vi "CAN Communication.vi"(8 "error in":errorcluster) -> (0 "error out":errorcluster)   [LabVIEW 2016]
uses:
  Typedefs/CAN Refnum.ctl
  Typedefs/CAN Session Pointer.ctl
  Typedefs/CAN Communication References.ctl
  Typedefs/kill process notifier array.ctl
  Typedefs/Write Queue.ctl
  Typedefs/FPGA CAN Frame Cluster.ctl
  <vilib>/userdefined/High Color/nirio_resource_hc.ctl
  <vilib>/FPGAPlugInAG/cRIO-9033/niLvFpga_Open_cRIO-9033.vi
  <vilib>/Utility/error.llb/Error Cluster From Error Code.vi
  <vilib>/RVI Host/nirviSupport.llb/nirviErrorClusterFromErrorCode.vi
  <vilib>/rvi/errors/niLvFpgaAdjustHostInterfaceError.vi
  <vilib>/FPGAPlugInAG/cRIO-9033/niLvFpga_Close_cRIO-9033.vi
  <vilib>/rvi/interface/nirviOpenFPGA/nirviOpenFPGA.xnode
  Users/s163601/Desktop/05-28/FPGA Bitfiles/project_FPGATarget_FPGAMain_boaNRF5GBP4.lvbitx
  Users/s163601/Desktop/05-28/FPGA Main.vi
  <vilib>/rvi/interface/nirviMethod/nirviMethod.xnode
  <vilib>/rvi/interface/nirviReadWriteControl/nirviReadWriteControl.xnode
  <vilib>/rvi/interface/nirviCloseFPGA/nirviCloseFPGA.xnode
  NiFpgaLv.dll
  <vilib>/rvi/interface/nirviMethod/StockFPGA_InlinedMethodWaitForSingleIRQ.vi
  <vilib>/FPGAPlugInAG/cRIO-9033/niLvFpga_WaitOnIrq_cRIO-9033.vi
  <vilib>/FPGAPlugInAG/cRIO-9033/niLvFpga_AcknowledgeIrq_cRIO-9033.vi
panel:
  out "CAN Session Out":T1
  in  "CAN Session In":T1
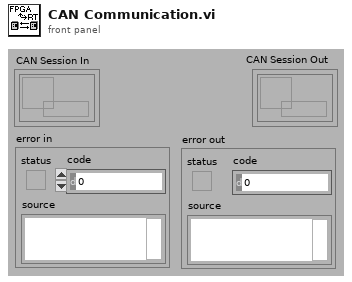
[diagram p1: front panel]
types:
  T1 = typedef "CAN Refnum.ctl" = refnum<k1>
  T2 = typedef "nirio_resource_hc.ctl" = tag
  T3 = typedef "kill process notifier array.ctl" = refnum<notifier>[]
  T4 = typedef "Write Queue.ctl" = refnum<queue>
  T5 = typedef "CAN Session Pointer.ctl" = refnum<queue>
  T6 = cluster{"Timestamp":u64, "Identifier":u32, "Type":u8, "InfoA":u8, "InfoB":u8, "DataLength":u8, "Data":u8[]}
  T7 = typedef "CAN Communication References.ctl" = cluster{"kill process notifier array":T3, "Write Queue":T4, "New Frame Notifier":refnum<notifier>, "Read Queue Array":T4[]}
  T8 = typedef "FPGA CAN Frame Cluster.ctl" = cluster{"Timestamp":u64, "Identifier":u32, "Type":u8, "InfoA":u8, "InfoB":u8, "DataLength":u8, "Data":u8[]}
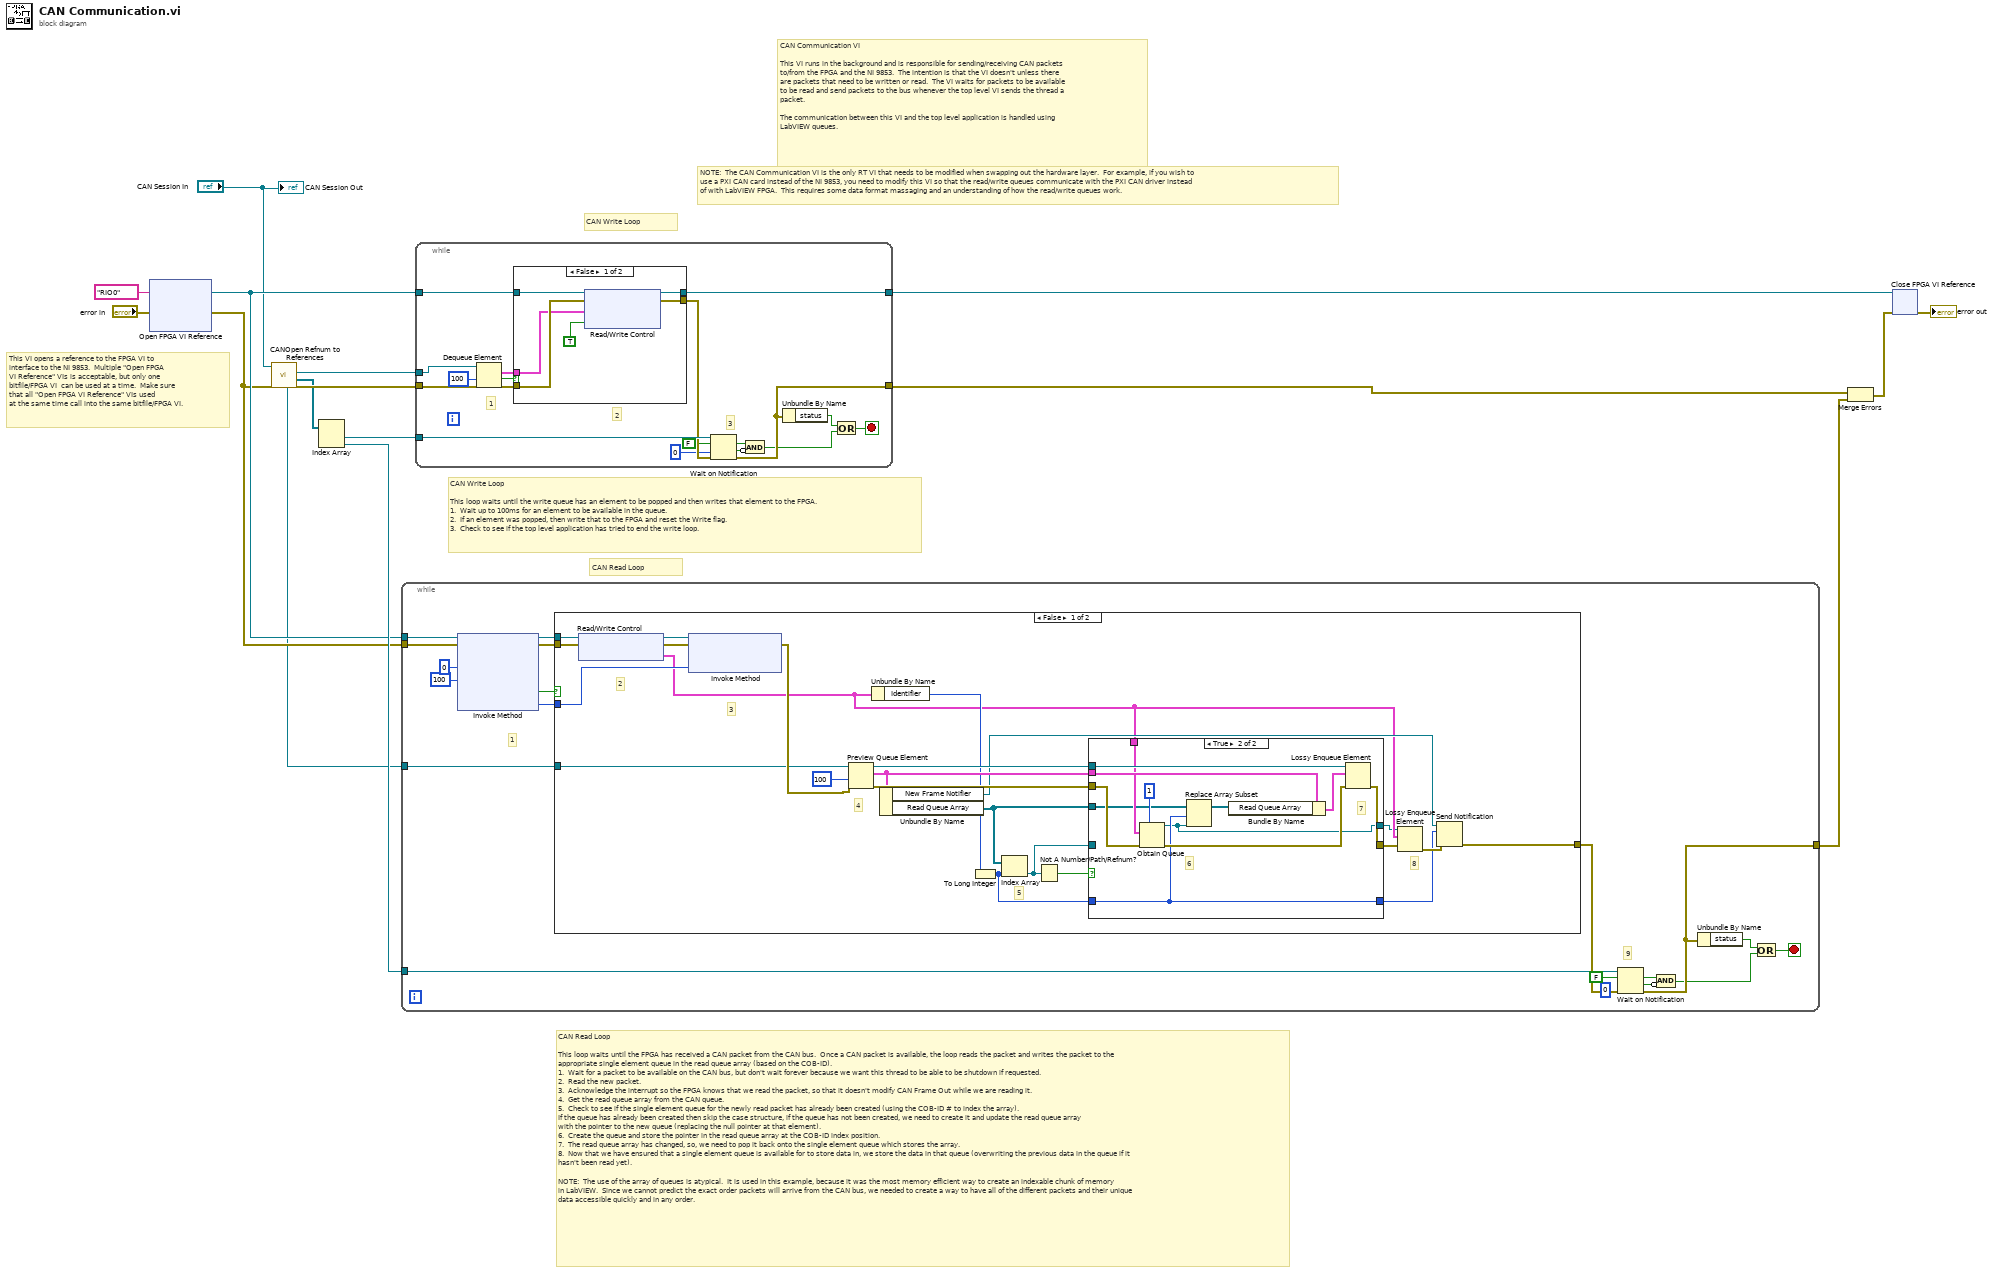
[diagram p0: block diagram]
diagram:
  # "This VI opens a reference to the FPGA VI to\ninterface to the NI 9853.  Multiple \"Open FPGA\nVI Reference\" VIs is acceptable, but only one\nbitfile/FPGA VI  can be used at a time.  Make sure\nthat all \"Open FPGA VI Reference\" VIs used\nat the same time call into the same bitfile/FPGA VI."
  # "NOTE:  The CAN Communication VI is the only RT VI that needs to be modified when swapping out the hardware layer.  For example, if you wish to\nuse a PXI CAN card instead of the NI 9853, you need to modify this VI so that the read/write queues communicate with the PXI CAN driver instead\nof with LabVIEW FPGA.  This requires some data format massaging and an understanding of how the read/write queues work."
  # "CAN Read Loop\n\nThis loop waits until the FPGA has received a CAN packet from the CAN bus.  Once a CAN packet is available, the loop reads the packet and writes the packet to the\nappropriate single element queue in the read queue array (based on the COB-ID).\n1.  Wait for a packet to be available on the CAN bus, but don't wait forever because we want this thread to be able to be shutdown if requested.\n2.  Read the new packet.\n3.  Acknowledge the interrupt so the FPGA knows that we read the packet, so that it doesn't modify CAN Frame Out while we are reading it.\n4.  Get the read queue array from the CAN queue.\n5.  Check to see if the single element queue for the newly read packet has already been created (using the COB-ID # to index the array).\nIf the queue has already been created then skip the case structure, if the queue has not been created, we need to create it and update the read queue array\nwith the pointer to the new queue (replacing the null pointer at that element).\n6.  Create the queue and store the pointer in the read queue array at the COB-ID index position.\n7.  The read queue array has changed, so, we need to pop it back onto the single element queue which stores the array.\n8.  Now that we have ensured that a single element queue is available for to store data in, we store the data in that queue (overwriting the previous data in the queue if it\nhasn't been read yet).\n\nNOTE:  The use of the array of queues is atypical.  It is used in this example, because it was the most memory efficient way to create an indexable chunk of memory\nin LabVIEW.  Since we cannot predict the exact order packets will arrive from the CAN bus, we needed to create a way to have all of the different packets and their unique\ndata accessible quickly and in any order."
  # "CAN Write Loop\n\nThis loop waits until the write queue has an element to be popped and then writes that element to the FPGA.\n1.  Wait up to 100ms for an element to be available in the queue.\n2.  If an element was popped, then write that to the FPGA and reset the Write flag.\n3.  Check to see if the top level application has tried to end the write loop."
  # "CAN Communication VI\n\nThis VI runs in the background and is responsible for sending/receiving CAN packets\nto/from the FPGA and the NI 9853.  The intention is that the VI doesn't unless there\nare packets that need to be written or read.  The VI waits for packets to be available\nto be read and send packets to the bus whenever the top level VI sends the thread a\npacket.\n\nThe communication between this VI and the top level application is handled using\nLabVIEW queues."
  # "CAN Read Loop"
  # "CAN Write Loop"
  n1 = xnode "Open FPGA VI Reference"("error in"="error in", "resource name"=T2 "RIO0") -> ("FPGA VI Reference Out"=w9:refnum<k20>, "error out"=w7:errorcluster)
  n2 = call "CANOpen Refnum to References.vi"("error in (no error)"=w7, "CAN Session In"="CAN Session In") -> ("error out"=w16:errorcluster, "kill process notifier array"=w13:T3, "Write Queue"=w15:T4, "CAN Session Queue"=w1:T5)  [unwired: 6 out]
  n3 = Index Array(array=w13) -> (element #1=w14:refnum<notifier>, element #2=w12:refnum<notifier>)  [unwired: 2 in]
  n4 = while {
    tunnel: w9 -> [w25]
    tunnel: w7 -> [w24]
    tunnel: [w32] -> w10
    tunnel: w12 -> [w28]
    tunnel: w1 -> [w17]
    stop <- w35 stop-if-true
    # "9"
    # "1"
    n5 = xnode "Invoke Method"("FPGA VI Reference In"=w25, "error in"=w24, "IRQ Number(s)"=0, "Timeout (ms)"=100) -> ("FPGA VI Reference Out"=w21:refnum<k20>, "error out"=w20:errorcluster, "Timed Out"=w19:bool, "IRQ(s) Asserted"=w18:i32)
    n6 = case shown="False" w19 {
      tunnel: w20 -> [w51 w74]
      tunnel: [w42 w74] -> w33
      tunnel: w21 -> [w52 _]
      tunnel: w18 -> [w48 _]
      tunnel: w17 -> [w46 _]
      frame False {
        # "8"
        # "5"
        # "4"
        # "3"
        # "2"
        n7 = xnode "Read/Write Control"("FPGA VI Reference In"=w52, "error in"=w51) -> ("FPGA VI Reference Out"=w50:refnum<k20>, "error out"=w49:errorcluster, "CAN Frame Out"=w40:T6)
        n8 = xnode "Invoke Method"("FPGA VI Reference In"=w50, "error in"=w49, "IRQ Number(s)"=w48) -> ("error out"=w47:errorcluster)  [unwired: 1 out]
        n9 = Preview Queue Element(queue=w46, timeout in ms (-1)=100, error in (no error)=w47) -> (queue out=w55:T5, element=w45:T7, error out=w56:errorcluster)  [unwired: 1 out]
        n10 = Unbundle By Name(w40) -> ("Identifier"=w41:u32)
        n11 = Unbundle By Name(w45) -> ("New Frame Notifier"=w44:refnum<notifier>, "Read Queue Array"=w36:T4[])
        n12 = To Long Integer(number=w41) -> (32bit integer=w53:i32)
        n13 = Index Array(array=w36, index=w53) -> (element=w37:T4)
        n14 = Not A Number/Path/Refnum?(number/path/refnum=w37) -> (NaN/Path/Refnum?=w58:bool)
        n15 = case shown="True" w58 {
          tunnel: w53 -> [w60 w65]
          tunnel: [w59 w62] -> w38
          tunnel: w56 -> [w61 w67]
          tunnel: [w61 w71] -> w57
          tunnel: w55 -> [_ w68]
          tunnel: w45 -> [_ w69]
          tunnel: w37 -> [w59 _]
          tunnel: w40 -> [_ w66]
          tunnel: [w60 w65] -> w39
          tunnel: w36 -> [_ w63]
          frame False {
          }
          frame True {
            # "7"
            # "6"
            n16 = Obtain Queue(max queue size (-1, unlimited)=1, element data type=w66, error in (no error)=w67) -> (queue out=w62:refnum<queue>, error out=w70:errorcluster)  [unwired: 1 in, 2 out]
            n17 = Replace Array Subset(array=w63, new element=w62, index=w65) -> (w64:T4[])
            n18 = Bundle By Name(cluster=w69, "Read Queue Array"=w64) -> (w72:T7)
            n19 = Lossy Enqueue Element(queue=w68, element=w72, error in (no error)=w70) -> (error out=w71:errorcluster)  [unwired: 3 out]
          }
        }
        n20 = Lossy Enqueue Element(queue=w38, element=w40, error in (no error)=w57) -> (error out=w43:errorcluster)  [unwired: 3 out]
        n21 = Send Notification(notification=w39, notifier=w44, error in (no error)=w43) -> (error out=w42:errorcluster)  [unwired: 1 out]
      }
      frame True {
      }
    }
    n22 = Wait on Notification(notifier=w28, ignore previous (F)=FALSE, timeout in ms (-1)=0, error in (no error)=w33) -> (notification=w31:bool, timed out?=w30:bool, error out=w32:errorcluster)  [unwired: 1 out]
    n23 = Compound Arithmetic op=AND(w31, invert w30) -> (w29:bool)
    n24 = Unbundle By Name(w32) -> ("status"=w34:bool)
    n25 = Or(x=w34, y=w29) -> (x .or. y?=w35:bool)
  }
  n26 = while {
    tunnel: w9 -> [w92]
    tunnel: [w81] -> w11
    tunnel: w16 -> [w89]
    tunnel: w15 -> [w84]
    tunnel: w14 -> [w83]
    tunnel: [w75] -> w6
    stop <- w91 stop-if-true
    # "3"
    # "2"
    # "1"
    n27 = Dequeue Element(queue=w84, timeout in ms (-1)=100, error in (no error)=w89) -> (element=w88:T8, timed out?=w85:bool, error out=w87:errorcluster)  [unwired: 1 out]
    n28 = case shown="False" w85 {
      tunnel: w92 -> [w97 w99]
      tunnel: [w96 w100] -> w82
      tunnel: w88 -> [w94 _]
      tunnel: w87 -> [w98 w100]
      tunnel: [w93 w99] -> w75
      frame False {
        n29 = xnode "Read/Write Control"("FPGA VI Reference In"=w97, "error in"=w98, "CAN Frame In"=w94, "Write"=TRUE) -> ("FPGA VI Reference Out"=w93:refnum<k20>, "error out"=w96:errorcluster)
      }
      frame True {
      }
    }
    n30 = Wait on Notification(notifier=w83, ignore previous (F)=FALSE, timeout in ms (-1)=0, error in (no error)=w82) -> (notification=w78:bool, timed out?=w77:bool, error out=w81:errorcluster)  [unwired: 1 out]
    n31 = Compound Arithmetic op=AND(w78, invert w77) -> (w76:bool)
    n32 = Unbundle By Name(w81) -> ("status"=w90:bool)
    n33 = Or(x=w90, y=w76) -> (x .or. y?=w91:bool)
  }
  n34 = Merge Errors(w11, w10) -> (w5:errorcluster)
  n35 = xnode "Close FPGA VI Reference"("FPGA VI Reference In"=w6, "error in"=w5) -> ("error out"=→"error out":errorcluster)
  "CAN Session Out" <- "CAN Session In"
